vi "WS1050 OFFSET CAL.vi"(8 "error in":errorcluster, 10 "OFFSET CAL":bool=TRUE) -> (0 "error out":errorcluster, 3 "AD7747 Values":string[][](table))   [LabVIEW 2012]
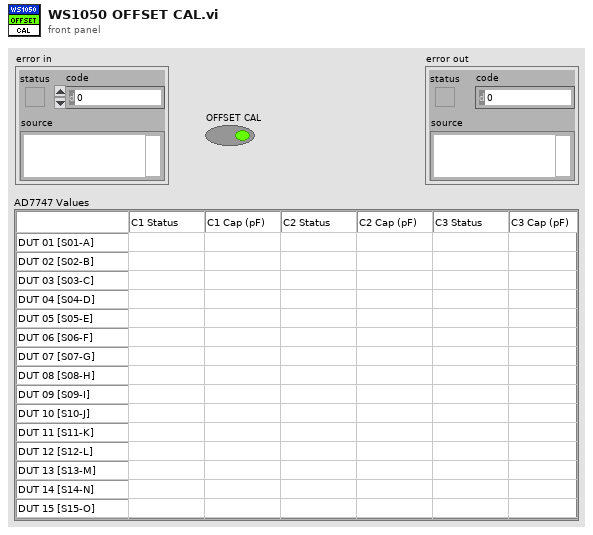
[diagram p1: front panel]
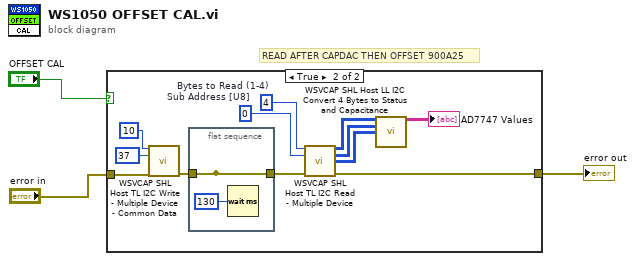
[diagram p0: block diagram]
diagram:
  # "READ AFTER CAPDAC THEN OFFSET 900A25"
  n1 = case shown="True" "OFFSET CAL" {
    tunnel: "error in" -> [w4 w16]
    tunnel: [w4 w5] -> w3
    frame False {
    }
    frame True {
      w11 = u8 4  # Bytes to Read (1-4)
      w12 = u8 0  # Sub Address [U8]
      n2 = call "WSVCAP SHL Host TL I2C Write - Multiple Device - Common Data.vi"("Sub Address"=u8 10, "Data Out [U8]"=u8 37, "error in"=w16) -> ("error out"=w13:errorcluster)  [unwired: 12 in]
      n3 = flat-sequence {
        tunnel: w13 -> [w17]
        tunnel: [w17] -> _
        tunnel: [w17] -> w6
        frame #0 {
          n4 = Wait (ms)(milliseconds to wait=u32 130) -> ()  [unwired: 1 out]
        }
      }
      n5 = call "WSVCAP SHL Host TL I2C Read - Multiple Device.vi"("Bytes to Read (1-4)"=w11, "Sub Address [U8]"=w12, "error in"=w6) -> ("C1:1-16 Read Data [U8]"=w10:u8[][], "C2:1-16 Read Data [U8]"=w9:u8[][], "C3:1-16 Read Data [U8]"=w7:u8[][], "error out"=w5:errorcluster)  [unwired: 9 in]
      n6 = call "WSVCAP SHL Host LL I2C Convert 4 Bytes to Status and Capacitance.vi"("C1:1-16 Read Data [U8]"=w10, "C2_1-16 Read Data [U8]"=w9, "C3_1-16 Read Data [U8]"=w7) -> ("AD7747 Values"=→"AD7747 Values":string[][])  [unwired: 12 in]
    }
  }
  "error out" <- w3
